vi "Pause.vi"(8 "error in (no error)":errorcluster, 11 "KNF Settings In":T1={"VISA resource name"="", "Simulated?"=TRUE}) -> (0 "error out":errorcluster, 1 "Connection Error":bool, 3 "KNF Settings Out":T1={"VISA resource name"="", "Simulated?"=TRUE})   [LabVIEW 2018, in "KNF SIMDOS.lvlib"]
uses:
  KNF SIMDOS.lvlib
  Settings Cluster plus SIMDOS.ctl
  <vilib>/KNF LAB/Driver S/Lvlib/SIMLAB_driver_lvclass/SIMLAB_driver.lvclass
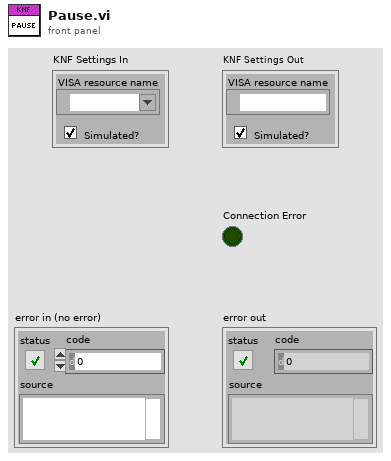
[diagram p1: front panel]
types:
  T1 = typedef "KNF SIMDOS.lvlib/Settings Cluster plus SIMDOS.ctl" = cluster{"VISA resource name":refnum<visa-resource-name>, "Simulated?":bool}
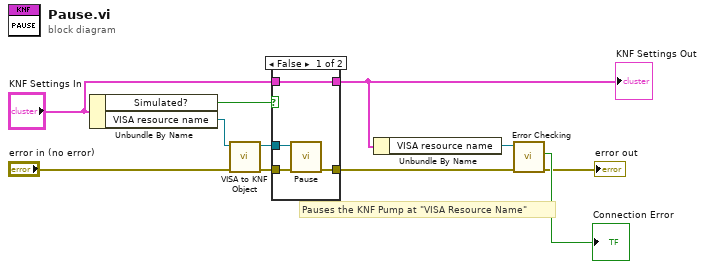
[diagram p0: block diagram]
diagram:
  # "Pauses the KNF Pump at \"VISA Resource Name\""
  n1 = Unbundle By Name("KNF Settings In") -> ("Simulated?"=w11:bool, "VISA resource name"=w7:refnum<visa-resource-name>)
  n2 = call "VISA to KNF Object.vi"("error in (no error)"="error in (no error)", "VISA resource name"=w7) -> ("error out"=w8:errorcluster, "SIMDOS out"=w6:refnum<class "SIMLAB_driver.lvclass">)  [unwired: 8 in]
  n3 = case shown="False" w11 {
    tunnel: [w14 w17] -> w4
    tunnel: w8 -> [w15 w17]
    tunnel: [w12 w16] -> w3
    tunnel: "KNF Settings In" -> [w12 w16]
    tunnel: w6 -> [w13 _]
    frame False {
      n4 = call <vilib>:"Pause.vi"("error in (no error)"=w15, "SIMDOS in"=w13) -> ("error out"=w14:errorcluster)  [unwired: 8 in, 1 out]
    }
    frame True {
    }
  }
  "KNF Settings Out" <- w3
  n5 = Unbundle By Name(w3) -> ("VISA resource name"=w2:refnum<visa-resource-name>)
  n6 = call "Error Checking.vi"("error in (no error)"=w4, "VISA resource name"=w2) -> ("error out"=→"error out":errorcluster, "Connection Error"=→"Connection Error":bool)  [unwired: 7 in, 1 out]
